vi "DT3120_InitDeviceList.vi"(8 "error in (no error)":errorcluster) -> (0 "error out":errorcluster, 2 "Alias List":string[](array[string]), 3 "Device List":T1(array[cluster]))   [LabVIEW 2010]
uses:
  Libs/olimg32.dll
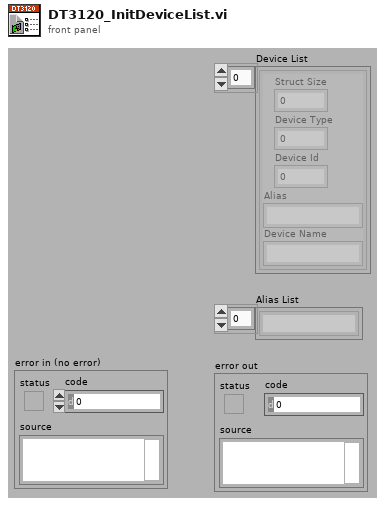
[diagram p1: front panel]
types:
  T1 = cluster{"Struct Size":u32, "Device Type":u32, "Device Id":u32, "Alias":string, "Device Name":string}[]
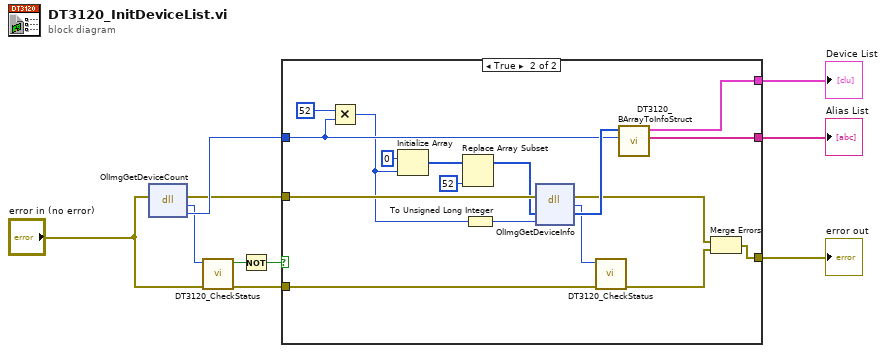
[diagram p0: block diagram]
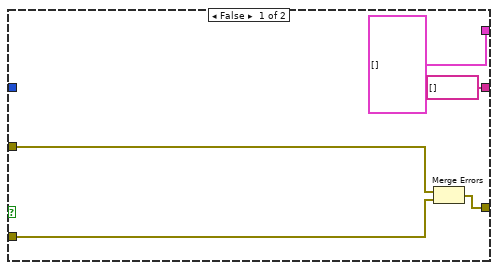
[diagram p2: hidden frame]
diagram:
  n1 = dll-call lib="C:/LabVIEW Programs/newMicroTime/Libs/olimg32.dll" fn="OlImgGetDeviceCount"(error in="error in (no error)") -> (error out=w1:errorcluster, "Status"=w2:u32, "iCount"=w5:i32)  [unwired: 2 in, 2 out]
  n2 = call "DT3120_CheckStatus.vi"("error in"="error in (no error)", "Status"=w2) -> ("error out"=w4:errorcluster, "New Error?"=w9:bool)  [unwired: 8 out]
  n3 = Not(x=w9) -> (.not. x?=w10:bool)
  n4 = case shown="True" w10 {
    tunnel: w1 -> [w13 w32]
    tunnel: w4 -> [w14 w30]
    tunnel: w5 -> [_ w27]
    tunnel: [string[] [] ("Alias List") w20] -> w6
    tunnel: [T1 [] ("Device List") w19] -> w7
    tunnel: [w15 w16] -> w8
    frame False {
      n5 = Merge Errors(w13, w14) -> (w15:errorcluster)
    }
    frame True {
      n6 = Multiply(x=52 ("ulListSize"), y=w27) -> (x*y=w21:i32)
      n7 = Initialize Array(u8 0 ("element"), w21) -> (w25:u8[])
      n8 = Replace Array Subset(array=w25, new element=u8 52 ("ulListSize")) -> (w23:u8[])  [unwired: 1 in]
      n9 = To Unsigned Long Integer(number=w21) -> (unsigned 32bit integer=w22:u32)
      n10 = dll-call lib="C:/LabVIEW Programs/newMicroTime/Libs/olimg32.dll" fn="OlImgGetDeviceInfo"(error in=w32, "lpDevList"=w23, "ulListSize"=w22) -> (error out=w18:errorcluster, "Status"=w29:u32, "lpDevList"=w31:u8[])  [unwired: 3 in, 1 out]
      n11 = call "DT3120_CheckStatus.vi"("error in"=w30, "Status"=w29) -> ("error out"=w17:errorcluster)  [unwired: 2 in, 7 out]
      n12 = call "DT3120_BArrayToInfoStruct.vi"("iCount"=w27, "lpDevList"=w31) -> ("Alias List"=w20:string[], "Device List"=w19:T1)  [unwired: 8 out]
      n13 = Merge Errors(w18, w17) -> (w16:errorcluster)
    }
  }
  "error out" <- w8
  "Device List" <- w7
  "Alias List" <- w6
